vi "sort2DArray.vi"(4 "index (row)":i32, 5 "Input Array":dbl[][](array[numeric])) -> (1 "Sorted Array":dbl[][](array[numeric]))   [LabVIEW 2012]
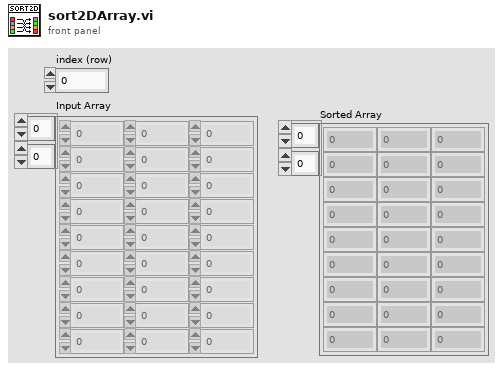
[diagram p1: front panel]
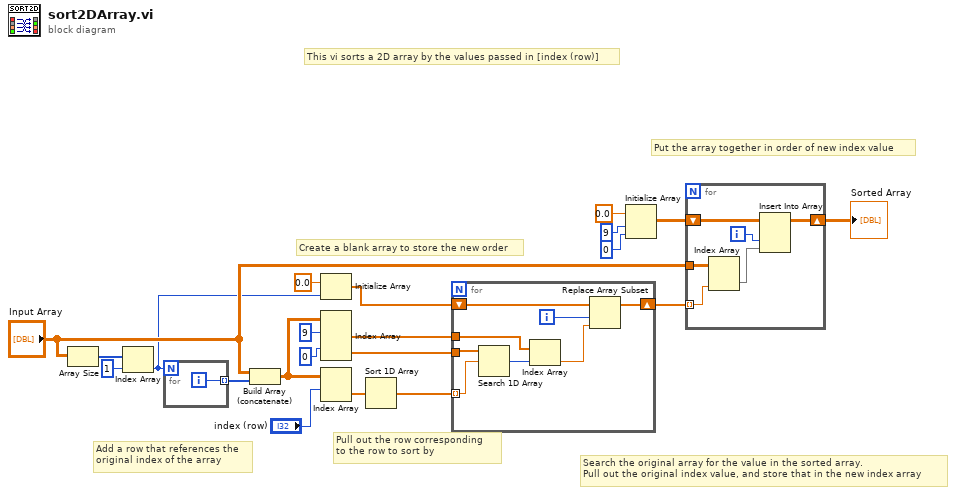
[diagram p0: block diagram]
diagram:
  # "This vi sorts a 2D array by the values passed in [index (row)]"
  # "Put the array together in order of new index value"
  # "Search the original array for the value in the sorted array.\nPull out the original index value, and store that in the new index array"
  # "Create a blank array to store the new order"
  # "Pull out the row corresponding\nto the row to sort by"
  # "Add a row that references the\noriginal index of the array"
  n1 = Array Size(array="Input Array") -> (size(s)=w9:i32[])
  n2 = Index Array(array=w9, index=1) -> (element=w1:i32)
  n3 = for {
    N: w1 -> [_]
    tunnel: [w22] -> w6 mode=indexing
    i -> [w22]
  }
  n4 = Build Array (concatenate)("Input Array", w6) -> (w5:dbl[][])
  n5 = Initialize Array(0.0 ("element"), w1) -> (w18:dbl[])
  n6 = Index Array(array=w5, index (row) #1=9 ("index (row)"), index (row) #2=0 ("disabled index (col)")) -> (element #1=w12:dbl[], element #2=w11:dbl[])  [unwired: 2 in]
  n7 = Index Array(array=w5, index (row)="index (row)") -> (element=w21:dbl[])  [unwired: 1 in]
  n8 = Sort 1D Array(array=w21) -> (sorted array=w20:dbl[])
  n9 = for {
    tunnel: w12 -> [w25]
    tunnel: w20 -> [w30] mode=indexing
    shift-right: [w28] -> w17
    shift-left: w18 -> [w27]
    tunnel: w11 -> [w26]
    i -> [w24]
    n10 = Search 1D Array(1D array=w26, element=w30) -> (index of element=w29:i32)  [unwired: 1 in]
    n11 = Index Array(array=w25, index=w29) -> (element=w23:dbl)
    n12 = Replace Array Subset(array=w27, new element=w23, index=w24) -> (w28:dbl[])
  }
  n13 = Initialize Array(0.0 ("element"), 9 ("dimension size"), 0 ("dimension size")) -> (w15:dbl[][])
  n14 = for {
    tunnel: w17 -> [w35] mode=indexing
    tunnel: "Input Array" -> [w36]
    shift-right: [w32] -> w4
    shift-left: w15 -> [w33]
    i -> [w31]
    n15 = Index Array(array=w36, index (col)=w35) -> (element=w34:dbl[])  [unwired: 1 in]
    n16 = Insert Into Array(array=w33, index (col)=w31, new element=w34) -> (w32:dbl[][])  [unwired: 1 in]
  }
  "Sorted Array" <- w4
